vi "Handle Last Ack Core.vi"(4 "error in (no error)":errorcluster, 6 "Last Ack":refnum<class "Last Ack.lvclass">, 7 "Guardian in":refnum<class "Guardian.lvclass">) -> (0 "error out":errorcluster, 3 "Guardian out":refnum<class "Guardian.lvclass">)   [LabVIEW 2026, in "TALOS.lvlib" / "Guardian.lvlib" / "Guardian.lvclass"]
doc: "(<B>Filename</B>: Actor Framework.lvlib:Actor.lvclass:Handle Last Ack Core.vi)\n\nDefines how the caller actor responds to the Last Ack message from a nested actor. The Last Ack message is the final message a nested actor sends to its caller before it shuts down. The message contains information about the final state of the nested actor.\n\nBy default, this method does nothing except return any error the nested actor sent. A descendant class may override this method to define behavior."
uses:
  Guardian.lvclass
  C:/LabVIEW Code/TALOS/talos/Ancestor/Ancestor/Ancestor.lvclass
  C:/LabVIEW Code/TALOS/builds/Actor Framework PPL/Actor Framework.lvlibp/1abvi3w/vi.lib/ActorFramework/Actor/Actor.lvclass
  builds/Actor Framework PPL/Actor Framework.lvlibp/1abvi3w/vi.lib/ActorFramework/LastAck/Last Ack.lvclass
  Ancestor/Ancestor/Ancestor.lvclass/Ancestor.ctl
  Guardian Messages/Broadcast to Guardians Msg/Broadcast to Guardians Msg.lvclass/Broadcast to Guardians Msg.ctl
  builds/Actor Framework PPL/Actor Framework.lvlibp/1abvi3w/vi.lib/ActorFramework/Message Enqueuer/Enqueue.vi
  Guardian Messages/Broadcast to Guardians Msg/Broadcast to Guardians Msg.lvclass
  Ancestor/Ancestor/Ancestor.lvclass
  builds/Actor Framework PPL/Actor Framework.lvlibp/1abvi3w/vi.lib/ActorFramework/Actor/Actor.lvclass
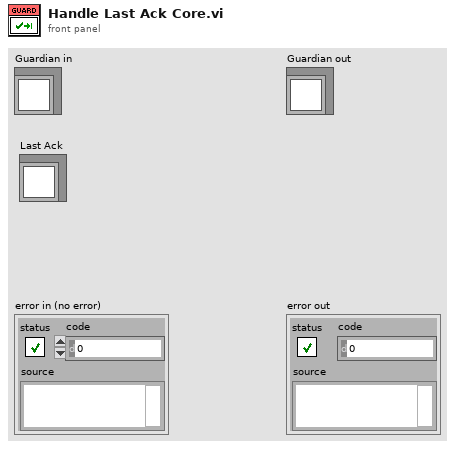
[diagram p1: front panel]
types:
  T1 = typedef "TALOS.lvlib/Classes.lvlib/uService List.lvclass/uService Properties.ctl" = cluster{"uService Queue":refnum<class "Message Enqueuer.lvclass">, "Last Pat":timestamp, "Online":bool, "Vi Ref":refnum<vi>, "Class name":string, "GUI":bool, "FP Items Refs Map":map{string, refnum<vi>}, "Remote GUI":bool, "Remote Window":refnum<vi>}
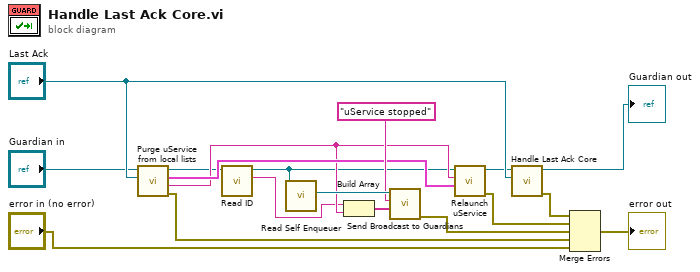
[diagram p0: block diagram]
diagram:
  n1 = call "Purge uService from local lists.vi"("Last Ack"="Last Ack", "Guardian in"="Guardian in") -> ("error out"=w5:errorcluster, "uService ID"=w4:string, "uService Properties"=w9:T1, "Guardian out"=w3:refnum<class "Guardian.lvclass">)  [unwired: 6 in]
  n2 = call "Read ID.vi"("Ancestor in"=w3) -> ("ID"=w1:string, "Ancestor out"=w2:refnum<class "Guardian.lvclass">)  [unwired: 8 in, 1 out]
  n3 = call "Read Self Enqueuer.vi"("Actor"=w2) -> ("Self Enqueuer"=w13:refnum<class "Message Enqueuer.lvclass">)  [unwired: 10 in]
  n4 = Build Array(w1, w4) -> (w11:string[])
  n5 = call "Send Broadcast to Guardians.vi"("Data"=w11, "Message"="uService stopped", "Message Enqueuer"=w13) -> ("error out"=w6:errorcluster)  [unwired: 7 in, 1 out]
  n6 = call "Relaunch uService.vi"("uService Properties"=w9, "uService ID"=w4, "Guardian in"=w2) -> ("error out"=w16:errorcluster, "Guardian out"=w8:refnum<class "Guardian.lvclass">)  [unwired: 7 in]
  n7 = call-parent "Handle Last Ack Core.vi"("Last Ack"="Last Ack", "Actor in"=w8) -> ("error out"=w7:errorcluster, "Actor out"=→"Guardian out":refnum<class "Guardian.lvclass">)  [unwired: 4 in]
  n8 = Merge Errors(w7, w16, w6, w5, "error in (no error)") -> (→"error out":errorcluster)
